vi "TypeDescriptor_GetRefClassName.vi"(10 "Ref Class":i16 format="%.0x") -> (2 "Reference Class":string)   [LabVIEW 2013, in "OpenDescriptor.lvlib"]
uses:
  OpenDescriptor.lvlib
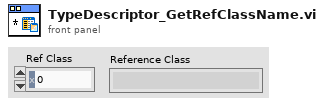
[diagram p1: front panel]
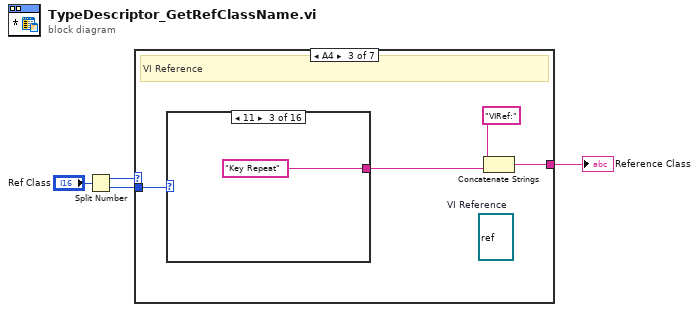
[diagram p0: block diagram]
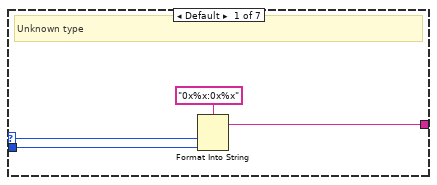
[diagram p2: hidden frame]
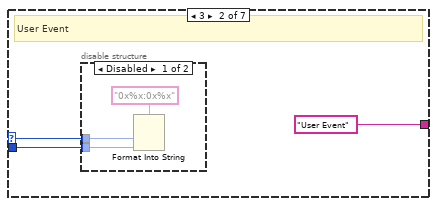
[diagram p3: hidden frame]
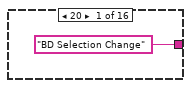
[diagram p5: hidden frame]
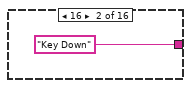
[diagram p6: hidden frame]
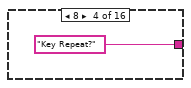
[diagram p7: hidden frame]
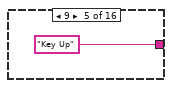
[diagram p8: hidden frame]
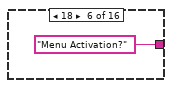
[diagram p9: hidden frame]
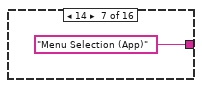
[diagram p10: hidden frame]
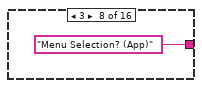
[diagram p11: hidden frame]
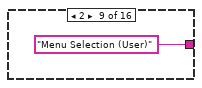
[diagram p12: hidden frame]
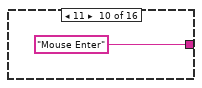
[diagram p13: hidden frame]
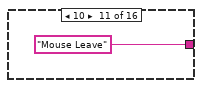
[diagram p14: hidden frame]
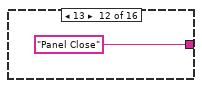
[diagram p15: hidden frame]
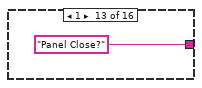
[diagram p16: hidden frame]
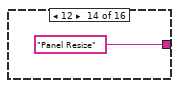
[diagram p17: hidden frame]
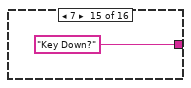
[diagram p18: hidden frame]
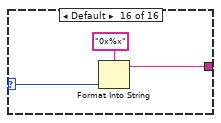
[diagram p19: hidden frame]
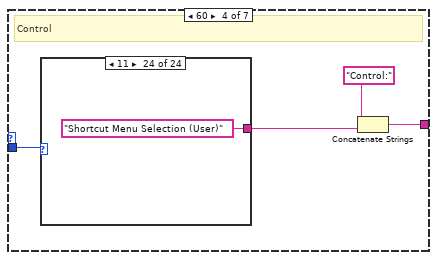
[diagram p20: hidden frame]
diagram:
  n1 = Split Number(x="Ref Class") -> (hi(x)=w1:u8, lo(x)=w2:u8)
  n2 = case shown="A4" w1 {
    selector: w1 -> [w7 w11 _ _ _ _ _]
    tunnel: w2 -> [w6 w10 w18 w38 w68 w85 w101]
    tunnel: [w5 "User Event" ("format string") w17 w40 w70 w87 w100] -> w3
    frame Default {
      # "Unknown type"
      n3 = Format Into String(format string="0x%x:0x%x", w7, w6) -> (resulting string=w5:string)  [unwired: 2 in, 1 out]
    }
    frame 3 {
      # "User Event"
      n4 = disable-structure shown="Disabled" {
        disable-tunnel: w11 -> [w13 _]
        disable-tunnel: w10 -> [w12 _]
        frame Disabled {
          n5 = Format Into String(format string="0x%x:0x%x", w13, w12) -> ()  [unwired: 2 in, 2 out]
        }
        frame Enabled {
        }
      }
    }
    frame 164 {
      (unwired) refnum<vi> refnum  # VI Reference
      # "VI Reference"
      n6 = case shown="11" w18 {
        selector: w18 -> [_ _ _ _ _ _ _ _ _ _ _ _ _ _ _ w35]
        tunnel: ["BD Selection Change" "Key Down" "Key Repeat" "Key Repeat?" "Key Up" "Menu Activation?" "Menu Selection (App)" "Menu Selection? (App)" "Menu Selection (User)" "Mouse Enter" "Mouse Leave" "Panel Close" "Panel Close?" "Panel Resize" "Key Down?" w36] -> w16
        frame 20 {
        }
        frame 16 {
        }
        frame 17 {
        }
        frame 8 {
        }
        frame 9 {
        }
        frame 18 {
        }
        frame 14 {
        }
        frame 3 {
        }
        frame 2 {
        }
        frame 11 {
        }
        frame 10 {
        }
        frame 13 {
        }
        frame 1 {
        }
        frame 12 {
        }
        frame 7 {
        }
        frame Default {
          n7 = Format Into String(format string="0x%x", w35) -> (resulting string=w36:string)  [unwired: 2 in, 1 out]
        }
      }
      n8 = Concatenate Strings("VIRef:" ("string"), w16) -> (w17:string)
    }
    frame 60 {
      # "Control"
      n9 = case shown="11" w38 {
        selector: w38 -> [w42 _ _ _ _ _ _ _ _ _ _ _ _ _ _ _ _ _ _ _ _ _ _ _]
        tunnel: [w41 "Value Change" "Drag Ended" "Drag Enter" "Drag Leave" "Drag Over" "Drag Source Update" "Drop" "Key Down" "Key Down?" "Key Repeat" "Key Repeat?" "Key Up" "Mouse Down" "Mouse Down?" "Mouse Enter" "Mouse Leave" "Mouse Move" "Mouse Up" "Mouse Wheel" "Shortcut Menu Activation?" "Shortcut Menu Selection? (App)" "Shortcut Menu Selection (App)" "Shortcut Menu Selection (User)"] -> w37
        frame Default {
          n10 = Format Into String(format string="0x%x", w42) -> (resulting string=w41:string)  [unwired: 2 in, 1 out]
        }
        frame 0 {
        }
        frame 14 {
        }
        frame 20 {
        }
        frame 22 {
        }
        frame 21 {
        }
        frame 15 {
        }
        frame 23 {
        }
        frame 10 {
        }
        frame 3 {
        }
        frame 11 {
        }
        frame 4 {
        }
        frame 5 {
        }
        frame 9 {
        }
        frame 1 {
        }
        frame 7 {
        }
        frame 8 {
        }
        frame 6 {
        }
        frame 2 {
        }
        frame 25 {
        }
        frame 16 {
        }
        frame 19 {
        }
        frame 18 {
        }
        frame 17 {
        }
      }
      n11 = Concatenate Strings("Control:" ("string"), w37) -> (w40:string)
    }
    frame 168 {
      # "Pane"
      n12 = case shown="8" w68 {
        selector: w68 -> [w72 _ _ _ _ _ _ _ _ _ _]
        tunnel: [w71 "Pane Size" "Shortcut Menu Activation?" "Shortcut Menu Selection (User)" "Mouse Down" "Mouse Down?" "Mouse Enter" "Mouse Leave" "Mouse Move" "Mouse Up" "Mouse Wheel"] -> w67
        frame Default {
          n13 = Format Into String(format string="0x%x", w72) -> (resulting string=w71:string)  [unwired: 2 in, 1 out]
        }
        frame 6 {
        }
        frame 7 {
        }
        frame 8 {
        }
        frame 5 {
        }
        frame 0 {
        }
        frame 3 {
        }
        frame 4 {
        }
        frame 2 {
        }
        frame 1 {
        }
        frame 9 {
        }
      }
      n14 = Concatenate Strings("Pane:" ("string"), w67) -> (w70:string)
    }
    frame 216 {
      # "Splitter"
      n15 = case shown="6" w85 {
        selector: w85 -> [w89 _ _ _ _ _ _ _]
        tunnel: [w88 "Mouse Down" "Mouse Down?" "Mouse Enter" "Mouse Leave" "Mouse Move" "Mouse Up" "Mouse Wheel"] -> w84
        frame Default {
          n16 = Format Into String(format string="0x%x", w89) -> (resulting string=w88:string)  [unwired: 2 in, 1 out]
        }
        frame 5 {
        }
        frame 0 {
        }
        frame 3 {
        }
        frame 4 {
        }
        frame 2 {
        }
        frame 1 {
        }
        frame 6 {
        }
      }
      n17 = Concatenate Strings("Splitter:" ("string"), w84) -> (w87:string)
    }
    frame 140 {
      (unwired) refnum<vi> refnum  # VI Reference
      # "Application Reference"
      n18 = case shown="5" w101 {
        selector: w101 -> [_ _ _ _ _ _ _ _ _ w112]
        tunnel: ["Application Activation" "Application Instance Close" "Application Instance Close?" "Bookmark Info Change" "Context Help Window Updated" "NI Security User Change" "VI Activation" "VI Deactivation" "VI Scroll" w113] -> w99
        frame 7 {
        }
        frame 2 {
        }
        frame 1 {
        }
        frame 14 {
        }
        frame 10 {
        }
        frame 6 {
        }
        frame 3 {
        }
        frame 15 {
        }
        frame 5 {
        }
        frame Default {
          n19 = Format Into String(format string="0x%x", w112) -> (resulting string=w113:string)  [unwired: 2 in, 1 out]
        }
      }
      n20 = Concatenate Strings("AppRef:" ("string"), w99) -> (w100:string)
    }
  }
  "Reference Class" <- w3
